vi "repeat cycle_exponential down.vi"(8 "error in (no error)":errorcluster caption="에러 입력(에러 없음)", 10 "waveform in":waveform(dbl), 11 "Waveform Obj 입력":refnum<class "PWL_DW7802.lvclass">) -> (0 "error out":errorcluster caption="에러 출력", 2 "waveform out":waveform(dbl), 3 "Waveform Obj 출력":refnum<class "PWL_DW7802.lvclass">)   [LabVIEW 2020, in "PWL_DW7802.lvclass"]
uses:
  PWL_DW7802.lvclass
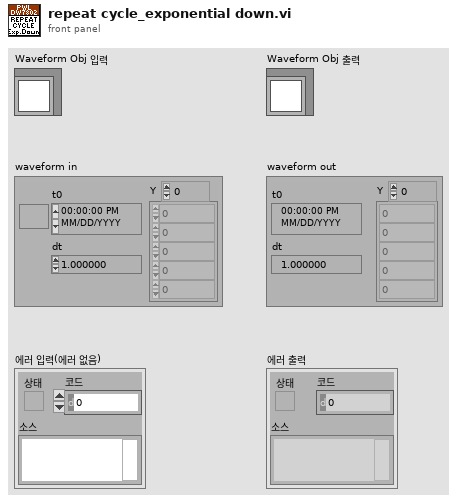
[diagram p1: front panel]
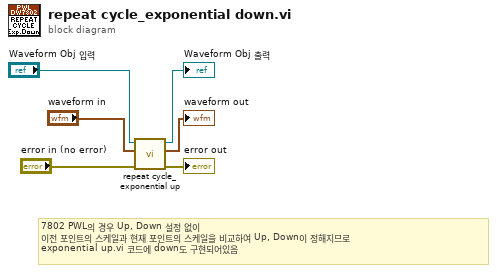
[diagram p0: block diagram]
diagram:
  # "7802 PWL의 경우 Up, Down 설정 없이\n이전 포인트의 스케일과 현재 포인트의 스케일을 비교하여 Up, Down이 정해지므로\nexponential up.vi 코드에 down도 구현되어있음"
  n1 = call-dynamic "repeat cycle_exponential up.vi"("error in (no error)"="error in (no error)", "waveform in"="waveform in", "Waveform Obj 입력"="Waveform Obj 입력") -> ("error out"=→"error out":errorcluster, "waveform out"=→"waveform out":waveform(dbl), "Waveform Obj 출력"=→"Waveform Obj 출력":refnum<class "PWL_DW7802.lvclass">)  [unwired: 6 in]
